vi "Momentum Killer.vi"(4 "Reverse Power":dbl, 5 "Edge":bool, 6 "Reverse Time (sec)":dbl, 7 "Stop Delay (sec)":dbl=0.5, 9 "Kill Control":bool, 11 "Power Input":dbl) -> (3 "Power Output":dbl)   [LabVIEW 2015]
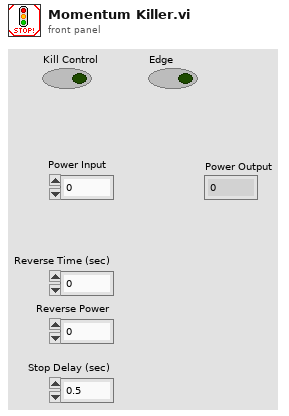
[diagram p1: front panel]
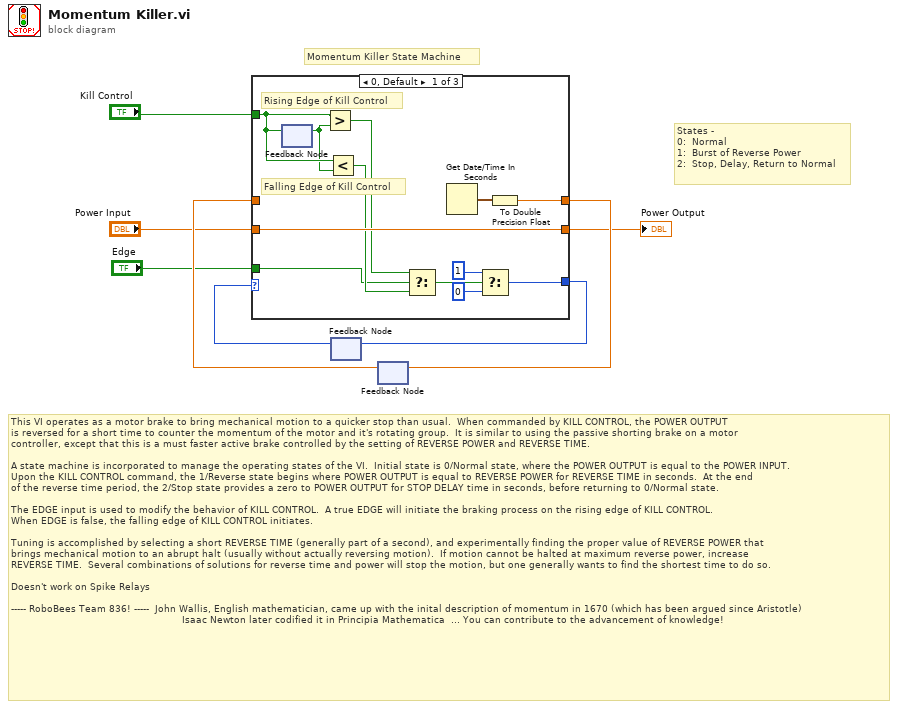
[diagram p0: block diagram]
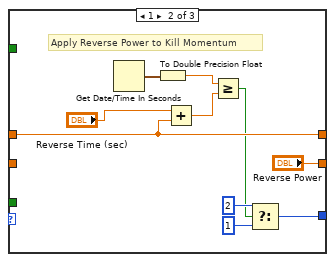
[diagram p2: hidden frame]
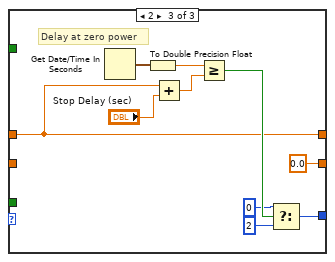
[diagram p3: hidden frame]
diagram:
  # "This VI operates as a motor brake to bring mechanical motion to a quicker stop than usual.  When commanded by KILL CONTROL, the POWER OUTPUT\nis reversed for a short time to counter the momentum of the motor and it's rotating group.  It is similar to using the passive shorting brake on a motor \ncontroller, except that this is a must faster active brake controlled by the setting of REVERSE POWER and REVERSE TIME.\n\nA state machine is incorporated to manage the operating states of the VI.  Initial state is 0/Normal state, where the POWER OUTPUT is equal to the POWER INPUT.\nUpon the KILL CONTROL command, the 1/Reverse state begins where POWER OUTPUT is equal to REVERSE POWER for REVERSE TIME in seconds.  At the end \nof the reverse time period, the 2/Stop state provides a zero to POWER OUTPUT for STOP DELAY time in seconds, before returning to 0/Normal state.\n\nThe EDGE input is used to modify the behavior of KILL CONTROL.  A true EDGE will initiate the braking process on the rising edge of KILL CONTROL.\nWhen EDGE is false, the falling edge of KILL CONTROL initiates.\n\nTuning is accomplished by selecting a short REVERSE TIME (generally part of a second), and experimentally finding the proper value of REVERSE POWER that \nbrings mechanical motion to an abrupt halt (usually without actually reversing motion).  If motion cannot be halted at maximum reverse power, increase \nREVERSE TIME.  Several combinations of solutions for reverse time and power will stop the motion, but one generally wants to find the shortest time to do so.\n\nDoesn't work on Spike Relays\n\n----- RoboBees Team 836! -----  John Wallis, English mathematician, came up with the inital description of momentum in 1670 (which has been argued since Aristotle)\n                                                         Isaac Newton later codified it in Principia Mathematica  ... You can contribute to the advancement of knowledge!"
  # "States - \n0:  Normal\n1:  Burst of Reverse Power\n2:  Stop, Delay, Return to Normal"
  # "Momentum Killer State Machine"
  n1 = feedback #1() -> (w6:i64)  [unwired: 1 in]
  n2 = feedback #2() -> (w8:dbl)  [unwired: 1 in]
  n3 = case shown="0, Default" w6 {
    tunnel: [w20 w28 w31] -> w5
    tunnel: "Kill Control" -> [w12 _ _]
    tunnel: "Power Input" -> [w17 _ _]
    tunnel: [w17 "Reverse Power" 0.0 ("FIRE")] -> w4
    tunnel: [w15 w26 w33] -> w7
    tunnel: w8 -> [_ w26 w33]
    tunnel: "Edge" -> [w9 _ _]
    frame 0, Default {
      # "Falling Edge of Kill Control"
      # "Rising Edge of Kill Control"
      n4 = feedback-in #3(w12) -> ()
      n5 = feedback #3() -> (w11:bool)  [unwired: 1 in]
      n6 = Greater?(x=w12, y=w11) -> (0:w14:bool)
      n7 = Less?(x=w12, y=w11) -> (x < y?=w10:bool)
      n8 = Select(t=w14, s=w9, f=w10) -> (s? t:f=w13:bool)
      n9 = Get Date/Time In Seconds() -> (seconds since 1Jan1904=w16:timestamp)
      n10 = Select(t=1, s=w13, f=0) -> (s? t:f=w20:i32)
      n11 = To Double Precision Float(number=w16) -> (double precision float=w15:dbl)
    }
    frame 1 {
      # "Apply Reverse Power to Kill Momentum"
      n12 = Get Date/Time In Seconds() -> (seconds since 1Jan1904=w30:timestamp)
      n13 = To Double Precision Float(number=w30) -> (double precision float=w25:dbl)
      n14 = Add(x="Reverse Time (sec)", y=w26) -> (x+y=w24:dbl)
      n15 = Greater Or Equal?(x=w25, y=w24) -> (x >= y?=w23:bool)
      n16 = Select(t=i64 2, s=w23, f=i64 1) -> (s? t:f=w28:i64)
    }
    frame 2 {
      # "Delay at zero power"
      n17 = Get Date/Time In Seconds() -> (seconds since 1Jan1904=w39:timestamp)
      n18 = To Double Precision Float(number=w39) -> (double precision float=w38:dbl)
      n19 = Add(x=w33, y="Stop Delay (sec)") -> (x+y=w37:dbl)
      n20 = Greater Or Equal?(x=w38, y=w37) -> (x >= y?=w36:bool)
      n21 = Select(t=0, s=w36, f=2) -> (s? t:f=w31:i32)
    }
  }
  "Power Output" <- w4
  n22 = feedback-in #1(w5) -> ()
  n23 = feedback-in #2(w7) -> ()
